vi "系统设置.vi"() -> ()   [LabVIEW 2016]
uses:
  <vilib>/Utility/miscctls.llb/LVPointTypeDef.ctl
  <vilib>/ptbypt/NI_PtbyPt.lvlib
  <vilib>/Utility/config.llb/NI_LVConfig.lvlib
  PLC/PLC.lvlib
panel:
  in  "更新":bool
  in  "updateconfiguration":T1={"主机"="27.154.58.30", "用户"="update", "密码"="std23506", "远程路径"="数据传输系统\\平台数据传输系统.exe", "下载文件名"="平台数据传输系统.exe", "软件版本"=""}
  in  "模块启用配置":bool
  in  "短信报警设置":bool
  in  "首页显示设置":bool
  in  "跨度核查":bool
  in  "空白核查":bool
  out "选项卡控件":enum32{"自由设定", "国标协议", "流量设定"}(tab)
  in  "24H周期设置":bool[](xcontrol)
  in  "运行间隔":i16=4 min=1 max=24
  in  "流量阈值":dbl=4.0 min=1.0 max=24.0
  in  "时间阈值":u16=4 min=1 max=24
  in  "周期设置":enum16{"自由设定", "国标协议", "流量设定"}(ring)
  out "x = y?":bool
  in  "质控启动日期":string(combo)="关闭"
  in  "跨度核查时间":u16(ring)=6 items=["00H", "01H", "02H", "03H", "04H", "05H", "06H", "07H", "08H", "09H", "10H", "11H", "12H", "13H", "14H", "15H", "16H", "17H", "18H", "19H", "20H", "21H", "22H", "23H", "关闭"]
  in  "空白核查时间":u16(ring)=2 items=["00H", "01H", "02H", "03H", "04H", "05H", "06H", "07H", "08H", "09H", "10H", "11H", "12H", "13H", "14H", "15H", "16H", "17H", "18H", "19H", "20H", "21H", "22H", "23H", "关闭"]
  in  "CODCr":bool
  in  "总磷总氮":bool
  in  "氨氮":bool
  in  "CODmn":bool
  in  "多参数":bool
  in  "输入密码":dbl
  in  "布尔":bool
  in  "副屏显示设置":bool
  in  "开机启动":bool caption="氨氮禁用"
  in  "运行模式":enum16{"维护模式", "常规模式", "应急模式", "质控模式"}(ring)
  # "注：周期设置分为自由设定和国标协议两种。\n1：选择自由设定情况下：运行间隔将不可选用并变灰色，周期设置可自由手动勾选\n2：选择国标协议情况下：周期时间将由运行间隔选择的时间决定，下方周期设置被禁用并无法手动勾选。\n3：选择流量设定情况下：瞬时流量连续超过流量阈值到达时间阈值设定值，仪器将自动开启测量。"
  # "自动运行启动参数"
  # "质控频次："
  # "空白核查时间："
  # "跨度核查时间："
  # "启动周期设置"
  # "m3/S"
  # "秒"
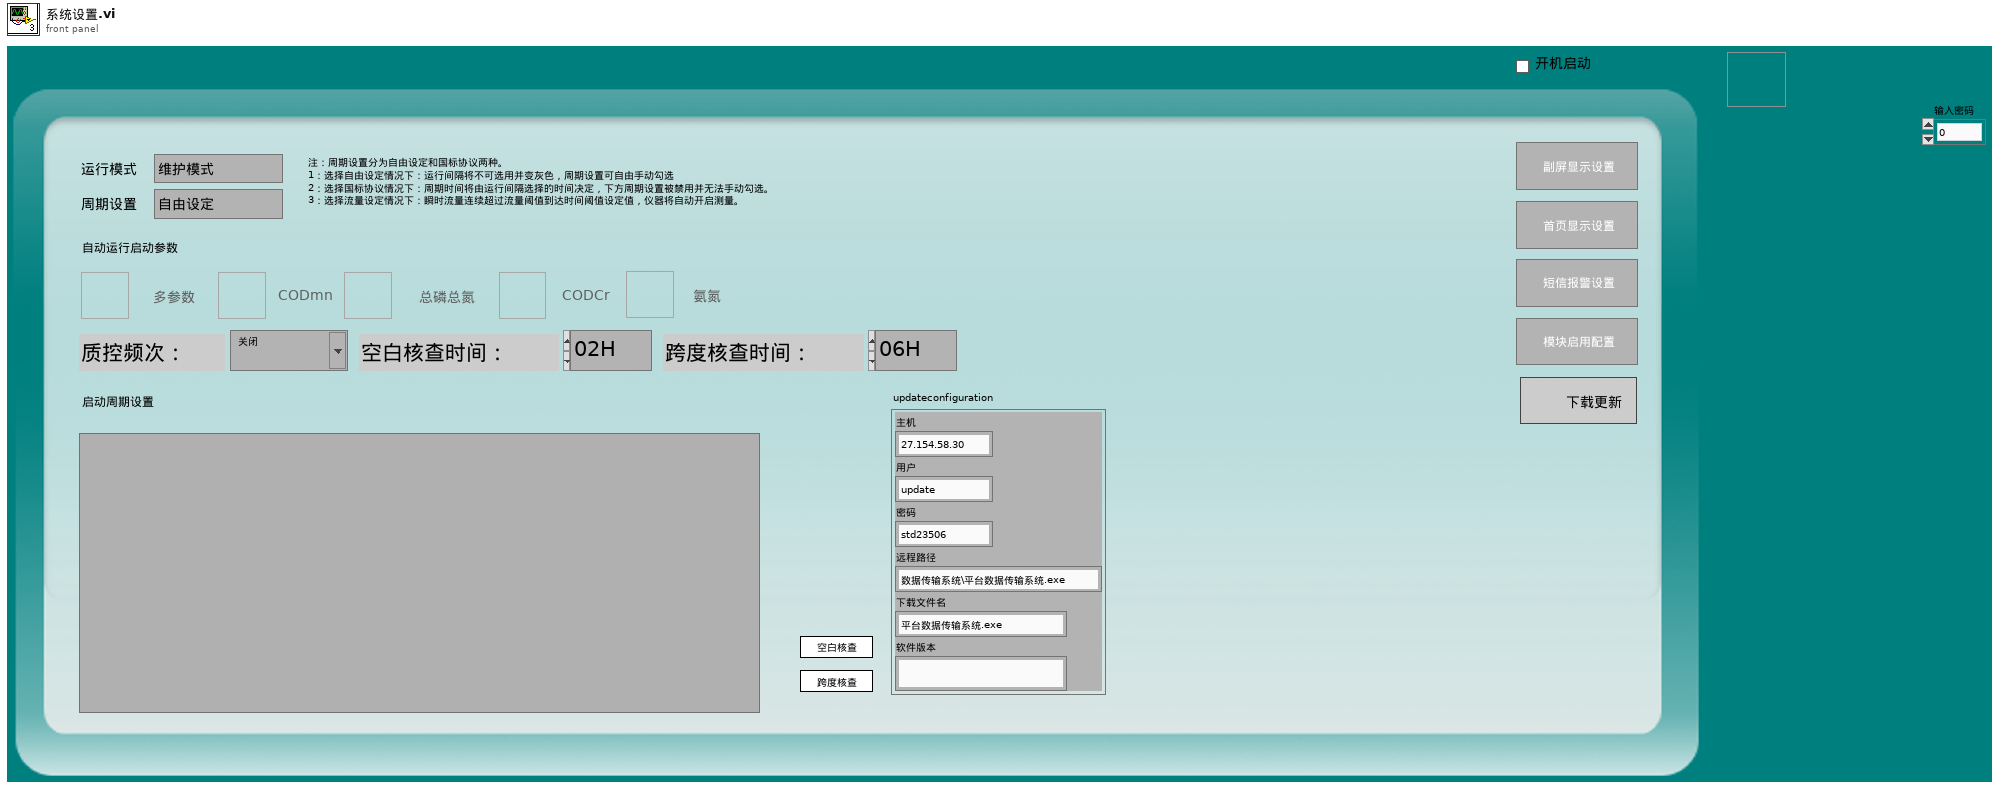
[diagram p1: front panel]
types:
  T1 = cluster{"主机":string, "用户":string, "密码":string, "远程路径":string, "下载文件名":string, "软件版本":string}
  T2 = typedef "NI_LVConfig.lvlib/Config Data RefNum.ctl" = refnum<k1>
  T3 = typedef "LVPointTypeDef.ctl" = cluster{"Horizontal":i16, "Vertical":i16}
  T4 = enum8{"Enabled", "Disabled", "Disabled and Grayed Out"}
  T5 = enum32{"Bad", "Idle", "Run top level", "Running"}
  T6 = enum32{"Invalid", "Standard", "Closed", "Hidden", "Minimized", "Maximized"}
  T7 = cluster{"运行模式":enum16{"维护模式", "常规模式", "应急模式", "质控模式"}}
  T8 = cluster{"测量模式":enum16{"水样测量", "标样核查", "零点核查", "跨度核查", "空白测试", "加标回收", "平行样", "校零", "校标"}}
  T9 = enum16{"启动测量", "标样核查", "零点核查", "跨度核查", "空白测试", "平行样测试", "加标回收", "空白校准", "标样校准", "初始化（清洗）", "停止测试", "仪器重启", "校时", "模式设置", "测量间隔设置"}
  T10 = cluster{"测试模式":enum16{"正常测试", "集成干预"}, "参数启用":cluster{"氨氮":bool, "总磷总氮":bool, "CODMn":bool, "CODcr":bool, "多参数":bool}}
  T11 = typedef "LVDateTimeRec.ctl" = cluster{"秒数的小数部分":dbl, "秒":i32, "分":i32, "时":i32, "日":i32, "月":i32, "年":i32, "天数（周）":i32, "天数（年）":i32, "DST":i32}
  T12 = cluster{"运行模式":enum16{"维护模式", "常规模式", "应急模式", "质控模式"}, "24H周期设置":bool[]}
  T13 = cluster{"运行模式":enum16{"维护模式", "常规模式", "应急模式", "质控模式"}, "质控频次":enum16{"关闭", "每天", "星期一", "星期二", "星期三", "星期四", "星期五", "星期六", "星期日"}, "空白核查时间":u16, "跨度核查时间":u16, "24H周期设置":bool[]}
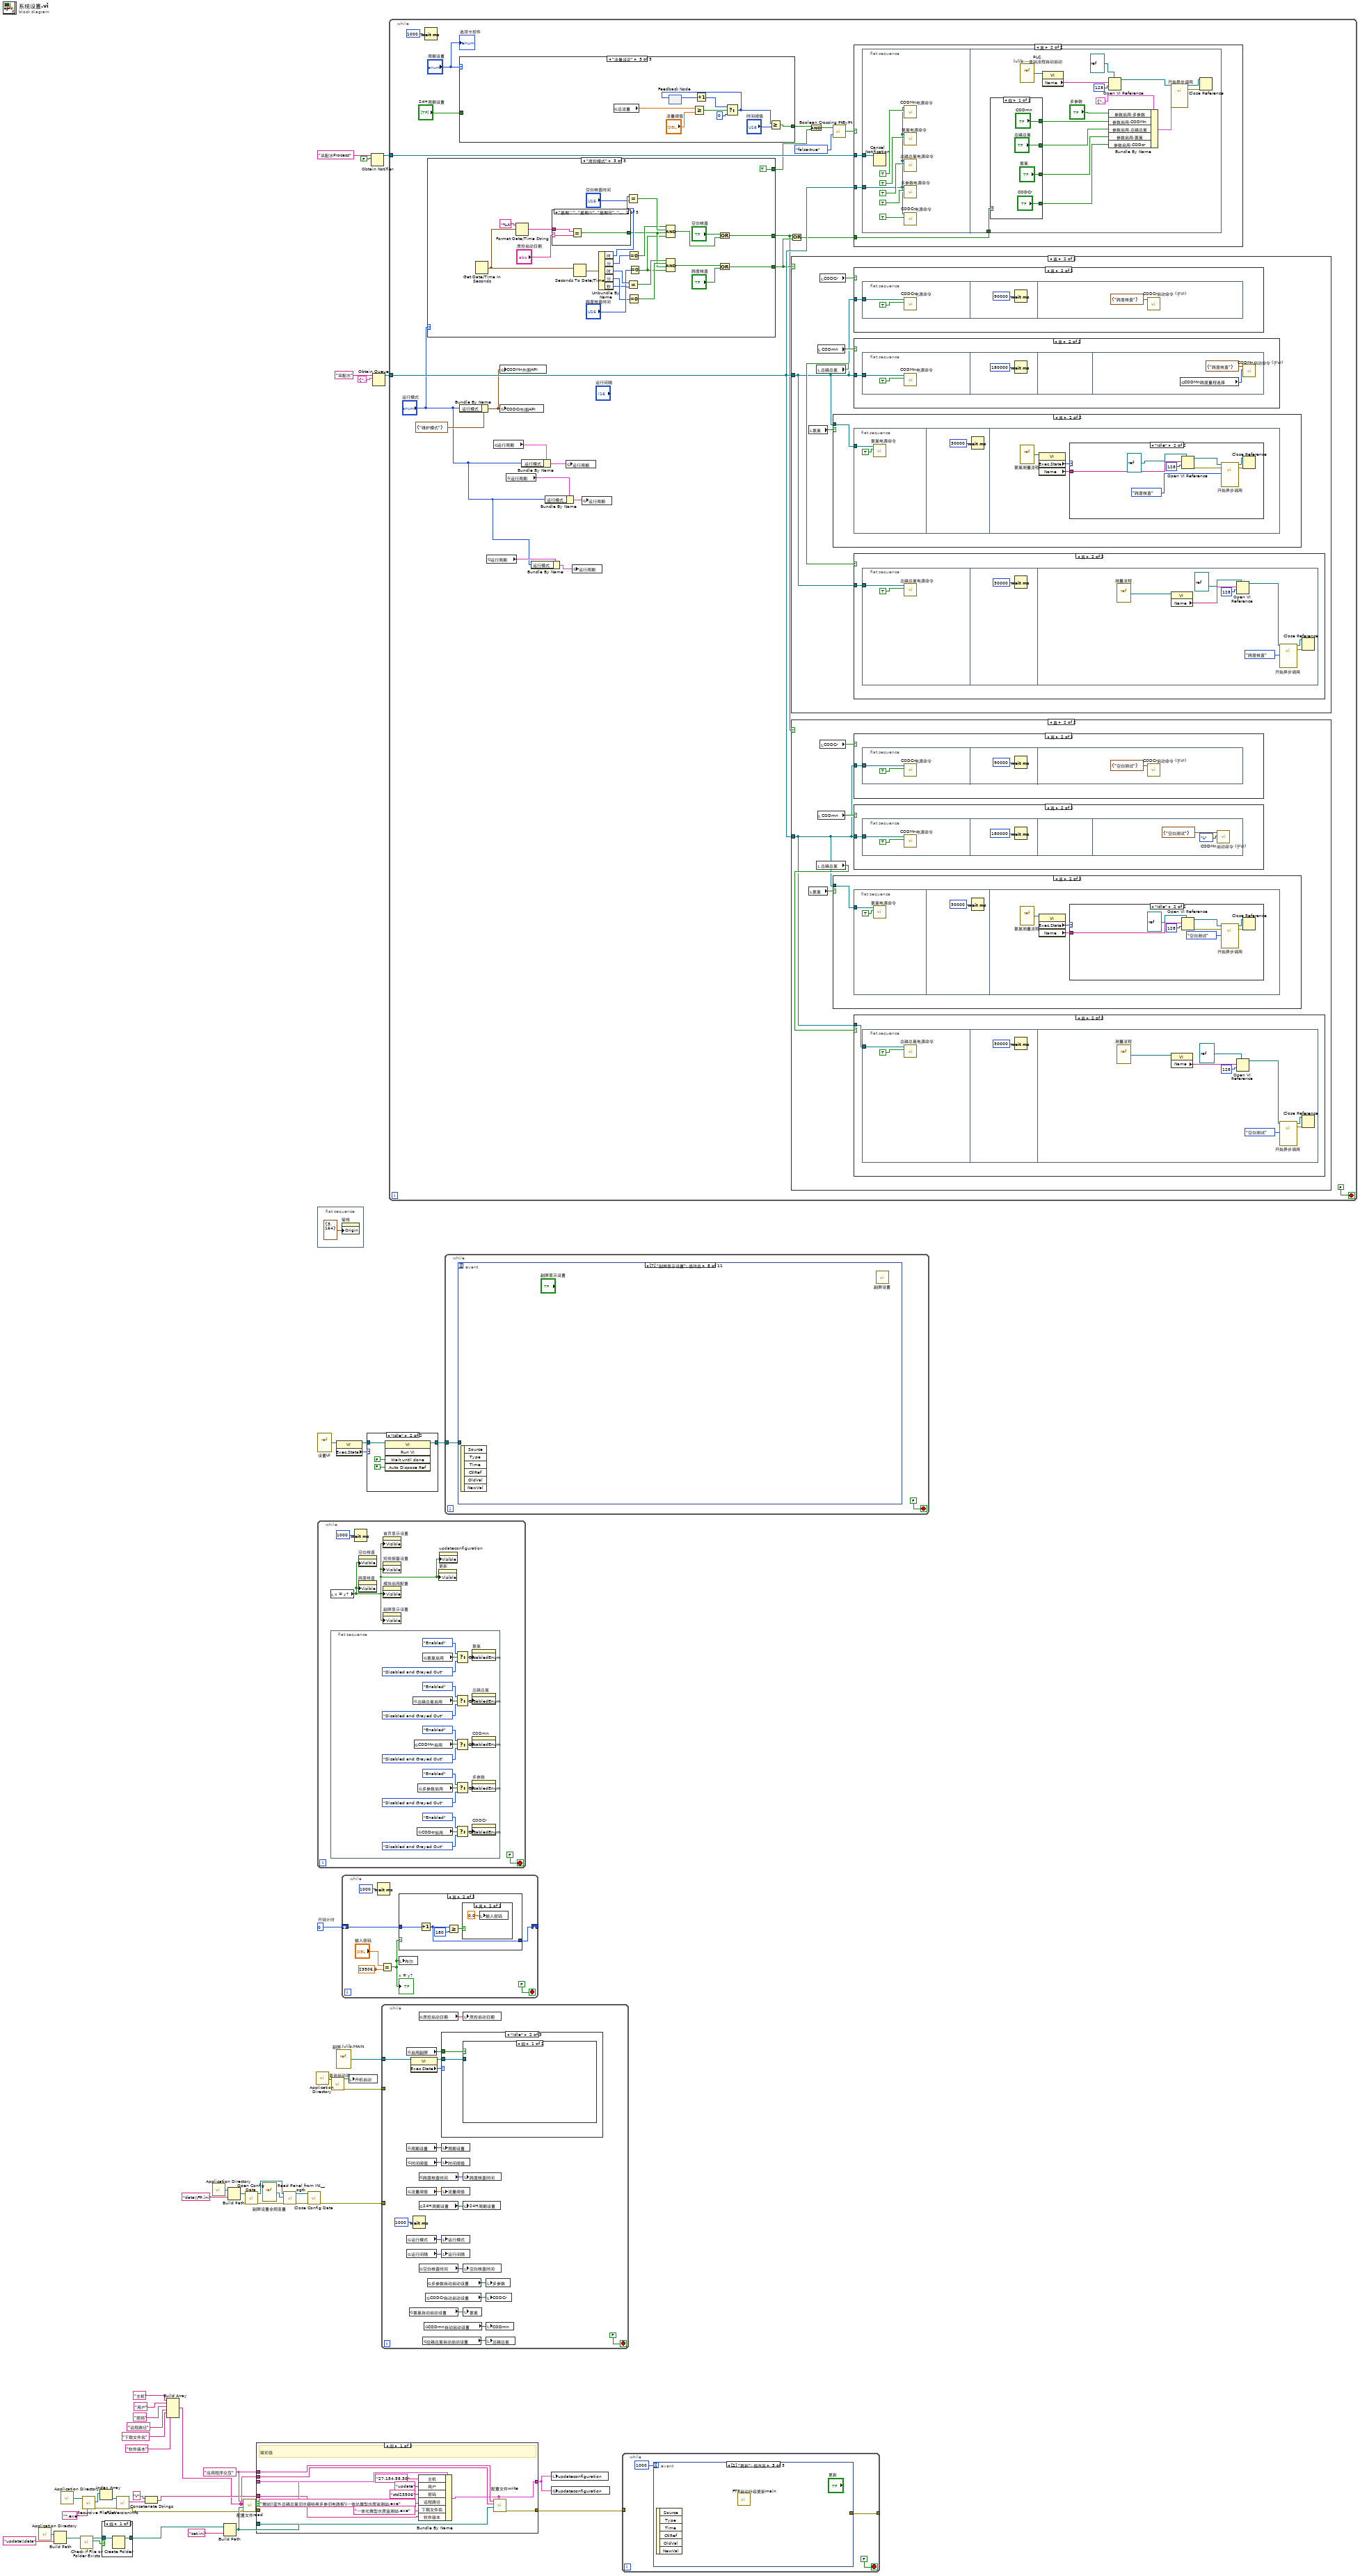
[diagram p0: block diagram]
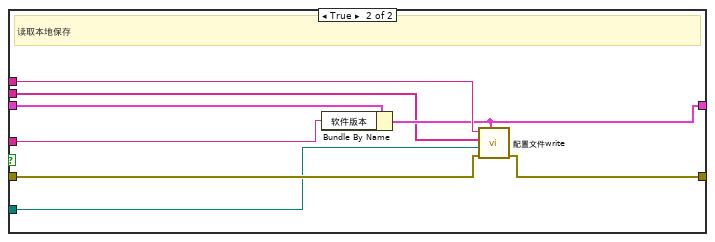
[diagram p3: hidden frame]
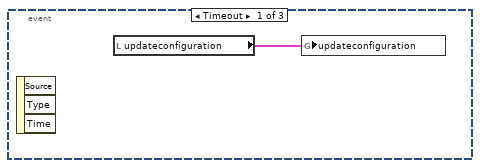
[diagram p4: hidden frame]
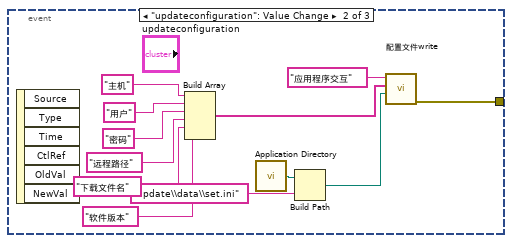
[diagram p5: hidden frame]
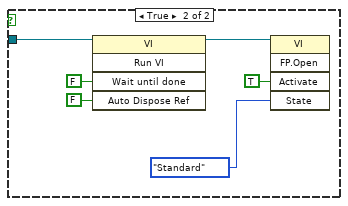
[diagram p10: hidden frame]
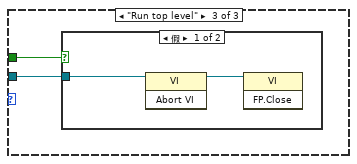
[diagram p11: hidden frame]
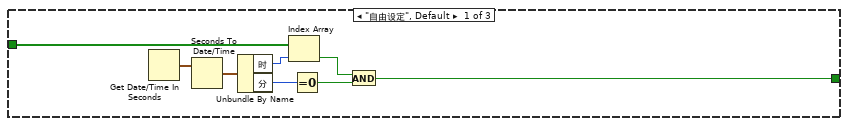
[diagram p13: hidden frame]
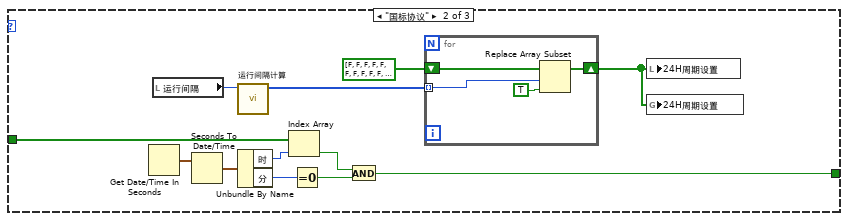
[diagram p14: hidden frame]
diagram:
  w28 = "应用程序交互" ("section")
  w49 = u32 0  # 开锁计时
  n1 = call <vilib>:"Application Directory.vi"() -> ("Application Directory"=w5:path)
  n2 = Build Path(base path=w5, name or relative path="update\\data" ("名称或相对路径")) -> (appended path=w6:path)
  n3 = call <vilib>:"Application Directory.vi"() -> ("Application Directory"=w23:path)
  n4 = call <vilib>:"Check if File or Folder Exists.vi"("path"=w6) -> ("file or folder exists?"=w7:bool, "dup path"=w8:path)  [unwired: 8 in, 1 out]
  n5 = call <vilib>:"Recursive File List.vi"("pattern"="*.exe", "Folder Path"=w23) -> ("error out"=w20:errorcluster, "All Files in Dir"=w22:path[])  [unwired: 5 in, 3 out]
  n6 = Index Array(array=w22) -> (element=w24:path)  [unwired: 1 in]
  n7 = case shown="假" w7 {
    tunnel: w8 -> [w56 w57]
    tunnel: [w55 w57] -> w3
    frame False {
      n8 = Create Folder(path (use dialog)=w56) -> (created path=w55:path)  [unwired: 2 in, 2 out]
    }
    frame True {
    }
  }
  n9 = call <vilib>:"FileVersionInfo.vi"("error in (no error)"=w20, "Application Path in"=w24) -> ("error out"=w17:errorcluster, "File Version Info"=w18:string)  [unwired: 6 in, 2 out]
  n10 = Concatenate Strings("V" ("字符串"), w18) -> (w16:string)
  n11 = Build Array("主机" ("section"), "用户" ("section"), "密码" ("key"), "远程路径" ("key"), "下载文件名" ("key"), "软件版本" ("key")) -> (w2:string[])
  n12 = call <vilib>:"Application Directory.vi"() -> ("Application Directory"=w31:path)
  n13 = Build Path(base path=w3, name or relative path="set.ini" ("名称或相对路径")) -> (appended path=w27:path)
  n14 = Build Path(base path=w31, name or relative path="data\\FP.ini" ("名称或相对路径")) -> (appended path=w38:path)
  n15 = call "配置文件read.vi"("error in (no error)"=w17, "configuration file path"=w27, "键数组"=w2, "段"=w28) -> ("error out"=w26:errorcluster, "section exists?"=w29:bool, "updateconfiguration"=w25:T1)  [unwired: 5 in]
  n16 = call <vilib>:"Open Config Data.vi"("configuration file path"=w38) -> ("error out"=w37:errorcluster, "refnum"=w34:T2)  [unwired: 8 in, 1 out]
  n17 = case shown="假" w29 {
    tunnel: w2 -> [w69 w73]
    tunnel: w28 -> [w68 w77]
    tunnel: w27 -> [w67 w71]
    tunnel: w26 -> [_ w72]
    tunnel: [w66 w70] -> w15
    tunnel: w25 -> [w60 w76]
    tunnel: [w58 w74] -> w1
    tunnel: w16 -> [w59 w75]
    frame False {
      # "赋初值"
      n18 = Bundle By Name(cluster=w60, "主机"="27.154.58.30" ("key"), "用户"="update", "密码"="std23506", "远程路径"="微站\\室外总磷总氮旧水箱哈希多参旧电路板\\一体化微型水质监测站.exe", "下载文件名"="一体化微型水质监测站.exe", "软件版本"=w59) -> (w58:T1)
      n19 = call "配置文件write.vi"("updateconfiguration"=w58, "configuration file path"=w67, "键数组"=w69, "段"=w68) -> ("error out"=w66:errorcluster)  [unwired: 7 in]
    }
    frame True {
      # "读取本地保存"
      n20 = Bundle By Name(cluster=w76, "软件版本"=w75) -> (w74:T1)
      n21 = call "配置文件write.vi"("updateconfiguration"=w74, "error in (no error)"=w72, "configuration file path"=w71, "键数组"=w73, "段"=w77) -> ("error out"=w70:errorcluster)  [unwired: 6 in]
    }
  }
  n22 = vi-ref "副屏设置全局变量.vi"() -> (w35:refnum<vi>)
  n23 = call <userlib>:"Read Panel from INI__ogtk.vi"("error in (no error)"=w37, "VI ref"=w35, "refnum"=w34) -> ("error out"=w36:errorcluster, "refnum out"=w33:T2)  [unwired: 7 in]
  n24 = call <vilib>:"Close Config Data.vi"("error in (no error)"=w36, "refnum"=w33) -> ("error out"=w32:errorcluster)  [unwired: 8 in, 1 out]
  n25 = call <vilib>:"Application Directory.vi"() -> ("Application Directory"=w51:path)
  n26 = flat-sequence {
    frame #0 {
      n27 = property on="窗格" class="Pane"("Origin"=T3 {"Horizontal"=3, "Vertical"=164} ("原点")) -> ()  [unwired: 2 in, 2 out]
    }
  }
  n28 = vi-ref "设置UI.vi"() -> (w44:refnum<vi>)
  n29 = while {
    stop <- FALSE stop-if-true
    n30 = local read "x = y?"() -> (w79:bool)
    n31 = flat-sequence {
      frame #0 {
        n32 = global read "系统设置全局变量.vi" "总磷总氮启用"() -> (w89:bool)
        n33 = global read "系统设置全局变量.vi" "CODMn启用"() -> (w87:bool)
        n34 = global read "系统设置全局变量.vi" "CODcr启用"() -> (w88:bool)
        n35 = global read "系统设置全局变量.vi" "多参数启用"() -> (w86:bool)
        n36 = global read "系统设置全局变量.vi" "氨氮启用"() -> (w82:bool)
        n37 = Select(t=T4."Enabled" ("禁用"), s=w82, f=T4."Disabled and Grayed Out" ("禁用")) -> (s? t:f=w90:T4)
        n38 = Select(t=T4."Enabled" ("禁用"), s=w89, f=T4."Disabled and Grayed Out" ("禁用")) -> (s? t:f=w84:T4)
        n39 = Select(t=T4."Enabled" ("禁用"), s=w87, f=T4."Disabled and Grayed Out" ("禁用")) -> (s? t:f=w91:T4)
        n40 = Select(t=T4."Enabled" ("禁用"), s=w86, f=T4."Disabled and Grayed Out" ("禁用")) -> (s? t:f=w85:T4)
        n41 = Select(t=T4."Enabled" ("禁用"), s=w88, f=T4."Disabled and Grayed Out" ("禁用")) -> (s? t:f=w101:T4)
        n42 = property on="氨氮" class="Bool (严格)"("DisabledEnum"=w90) -> ()  [unwired: 2 in, 2 out]
        n43 = property on="总磷总氮" class="Bool (严格)"("DisabledEnum"=w84) -> ()  [unwired: 2 in, 2 out]
        n44 = property on="CODmn" class="Bool (严格)"("DisabledEnum"=w91) -> ()  [unwired: 2 in, 2 out]
        n45 = property on="多参数" class="Bool (严格)"("DisabledEnum"=w85) -> ()  [unwired: 2 in, 2 out]
        n46 = property on="CODCr" class="Bool (严格)"("DisabledEnum"=w101) -> ()  [unwired: 2 in, 2 out]
      }
    }
    n47 = Wait (ms)(milliseconds to wait=u32 1000 ("等待时间（毫秒）")) -> ()  [unwired: 1 out]
    n48 = property on="空白核查" class="Bool"("Visible"=w79) -> ()  [unwired: 2 in, 2 out]
    n49 = property on="跨度核查" class="Bool"("Visible"=w79) -> ()  [unwired: 2 in, 2 out]
    n50 = property on="首页显示设置" class="Bool"("Visible"=w79) -> ()  [unwired: 2 in, 2 out]
    n51 = property on="短信报警设置" class="Bool"("Visible"=w79) -> ()  [unwired: 2 in, 2 out]
    n52 = property on="模块启用配置" class="Bool"("Visible"=w79) -> ()  [unwired: 2 in, 2 out]
    n53 = property on="副屏显示设置" class="Bool"("Visible"=w79) -> ()  [unwired: 2 in, 2 out]
    n54 = property on="更新" class="Bool"("Visible"=w79) -> ()  [unwired: 2 in, 2 out]
    n55 = property on="updateconfiguration" class="Clust (严格)"("Visible"=w79) -> ()  [unwired: 2 in, 2 out]
  }
  n56 = call "查询启动项.vi"("启动文件路径"=w51) -> ("error out"=w40:errorcluster, "包含启动项"=w50:bool)  [unwired: 9 in]
  n57 = property class="VI"(reference=w44) -> (reference out=w42:refnum<vi>, "Exec.State"=w43:T5)  [unwired: 1 in, 1 out]
  n58 = vi-ref "副屏.lvlib:MAIN.vi"() -> (w45:refnum<vi>)
  n59 = while {
    shift-right: [w103] -> _
    shift-left: w49 -> [w104]
    stop <- FALSE stop-if-true
    n60 = Wait (ms)(milliseconds to wait=u32 1000 ("等待时间（毫秒）")) -> ()  [unwired: 1 out]
    n61 = Equal?(x="输入密码", y=23506.0) -> (x = y?=w102:bool)
    "x = y?" <- w102
    n62 = case shown="真" w102 {
      tunnel: w104 -> [_ w112]
      tunnel: [_ w111] -> w103
      frame False {
      }
      frame True {
        n63 = Increment(x=w112) -> (x+1=w111:u32)
        n64 = Greater Or Equal?(x=w111, y=u32 180) -> (x >= y?=w109:bool)
        n65 = case shown="真" w109 {
          frame False {
          }
          frame True {
            n66 = local write "输入密码"(0.0 ("输入密码")) -> ()
          }
        }
      }
    }
    n67 = local write "布尔"(w102) -> ()
  }
  n68 = local write "开机启动"(w50) -> ()
  n69 = case shown="\"Idle\"" w43 {
    tunnel: w42 -> [w114 w118]
    tunnel: [w114 w117] -> w41
    frame "Bad", Default {
    }
    frame "Idle" {
      n70 = invoke class="VI" method="Run VI"(reference=w118, "Wait until done"=FALSE ("结束前等待"), "Auto Dispose Ref"=FALSE ("自动销毁引用")) -> (reference out=w117:refnum<vi>)  [unwired: 2 in, 4 out]
    }
  }
  n71 = Obtain Notifier(name (unnamed)="采配水Process" ("名称（未命名）"), notification data type=FALSE) -> (notifier out=w52:refnum<notifier>)  [unwired: 2 in, 2 out]
  n72 = Obtain Queue(name (unnamed)="采配水" ("名称（未命名）"), element data type=cluster{"命令":string, "数据":variant} {"命令"="", "数据"=variant}) -> (queue out=w46:refnum<queue>)  [unwired: 3 in, 2 out]
  n73 = while {
    tunnel: w45 -> [w130]
    tunnel: w40 -> [_]
    tunnel: w32 -> [_]
    stop <- FALSE stop-if-true
    n74 = global read "副屏设置全局变量.vi" "启用副屏"() -> (w128:bool)
    n75 = global read "系统设置全局变量.vi" "周期设置"() -> (w123:enum16{"自由设定", "国标协议", "流量设定"})
    n76 = global read "系统设置全局变量.vi" "时间阈值"() -> (w119:u16)
    n77 = global read "系统设置全局变量.vi" "流量阈值"() -> (w120:dbl)
    n78 = global read "系统设置全局变量.vi" "运行模式"() -> (w121:enum16{"维护模式", "常规模式", "应急模式", "质控模式"})
    n79 = global read "系统设置全局变量.vi" "运行间隔"() -> (w122:i16)
    n80 = global read "系统设置全局变量.vi" "氨氮自动启动设置"() -> (w135:bool)
    n81 = property class="VI"(reference=w130) -> (reference out=w127:refnum<vi>, "Exec.State"=w129:T5)  [unwired: 1 in, 1 out]
    n82 = Wait (ms)(milliseconds to wait=u32 1000 ("等待时间（毫秒）")) -> ()  [unwired: 1 out]
    n83 = global read "系统设置全局变量.vi" "质控启动日期"() -> (w126:string)
    n84 = global read "系统设置全局变量.vi" "跨度核查时间"() -> (w124:u16)
    n85 = global read "系统设置全局变量.vi" "24H周期设置"() -> (w136:bool[])
    n86 = global read "系统设置全局变量.vi" "空白核查时间"() -> (w125:u16)
    n87 = global read "系统设置全局变量.vi" "总磷总氮自动启动设置"() -> (w133:bool)
    n88 = global read "系统设置全局变量.vi" "CODmn自动启动设置"() -> (w132:bool)
    n89 = global read "系统设置全局变量.vi" "CODCr自动启动设置"() -> (w134:bool)
    n90 = global read "系统设置全局变量.vi" "多参数自动启动设置"() -> (w131:bool)
    n91 = case shown="\"Idle\"" w129 {
      tunnel: w128 -> [_ w139 w147]
      tunnel: w127 -> [_ w140 w148]
      frame "Bad", Default {
      }
      frame "Idle" {
        n92 = case shown="假" w139 {
          tunnel: w140 -> [_ w146]
          frame False {
          }
          frame True {
            n93 = invoke class="VI" method="Run VI"(reference=w146, "Wait until done"=FALSE ("结束前等待"), "Auto Dispose Ref"=FALSE ("自动销毁引用")) -> (reference out=w141:refnum<vi>)  [unwired: 2 in, 4 out]
            n94 = invoke class="VI" method="FP.Open"(reference=w141, "Activate"=TRUE ("激活？"), "State"=T6."Standard" ("状态")) -> ()  [unwired: 2 in, 5 out]
          }
        }
      }
      frame "Run top level" {
        n95 = case shown="假" w147 {
          tunnel: w148 -> [w149 _]
          frame False {
            n96 = invoke class="VI" method="Abort VI"(reference=w149) -> (reference out=w150:refnum<vi>)  [unwired: 2 in, 2 out]
            n97 = invoke class="VI" method="FP.Close"(reference=w150) -> ()  [unwired: 2 in, 3 out]
          }
          frame True {
          }
        }
      }
    }
    n98 = local write "周期设置"(w123) -> ()
    n99 = local write "时间阈值"(w119) -> ()
    n100 = local write "流量阈值"(w120) -> ()
    n101 = local write "运行模式"(w121) -> ()
    n102 = local write "运行间隔"(w122) -> ()
    n103 = local write "质控启动日期"(w126) -> ()
    n104 = local write "跨度核查时间"(w124) -> ()
    n105 = local write "24H周期设置"(w136) -> ()
    n106 = local write "空白核查时间"(w125) -> ()
    n107 = local write "氨氮"(w135) -> ()
    n108 = local write "多参数"(w131) -> ()
    n109 = local write "CODCr"(w134) -> ()
    n110 = local write "CODmn"(w132) -> ()
    n111 = local write "总磷总氮"(w133) -> ()
  }
  n112 = while {
    tunnel: w52 -> [w171]
    tunnel: w46 -> [w167]
    stop <- FALSE stop-if-true
    n113 = Wait (ms)(milliseconds to wait=u32 1000 ("等待时间（毫秒）")) -> ()  [unwired: 1 out]
    n114 = case shown="\"质控模式\"" "运行模式" {
      tunnel: [_ _ w323] -> w161
      tunnel: [_ _ w327] -> w160
      tunnel: [_ TRUE TRUE] -> w164
      frame "维护模式", Default {
      }
      frame "常规模式" {
      }
      frame "质控模式" {
        n115 = Get Date/Time In Seconds() -> (seconds since 1Jan1904=w334:timestamp)
        n116 = Format Date/Time String(time format string (%c)="%A" ("时间格式字符串(%c)"), seconds (now)=w334) -> (date/time string=w332:string)  [unwired: 1 in]
        n117 = case shown="\"星期二\", \"星期六\", \"星期日\", \"星期三\", \"星期四\", \"星期五\", \"星期一\"" "质控启动日期" {
          selector: "质控启动日期" -> [w350 _ _]
          tunnel: [w349 TRUE FALSE] -> w335
          tunnel: w332 -> [w348 _ _]
          frame "星期二", "星期六", "星期日", "星期三", "星期四", "星期五", "星期一" {
            n118 = Equal?(x=w348, y=w350) -> (x = y?=w349:bool)
          }
          frame "每天" {
          }
          frame "关闭", Default {
          }
        }
        n119 = Seconds To Date/Time(time stamp (now)=w334) -> (date time rec=w347:T11)  [unwired: 1 in]
        n120 = Unbundle By Name(w347) -> ("时"=w346:i32, "分"=w344:i32, "时"=w340:i32, "分"=w339:i32, "秒"=w331:i32)
        n121 = Equal?(x=w346, y="空白核查时间") -> (x = y?=w343:bool)
        n122 = Equal?(x=w340, y="跨度核查时间") -> (x = y?=w338:bool)
        n123 = Equal To 0?(x=w344) -> (x = 0?=w342:bool)
        n124 = Equal To 0?(x=w339) -> (x = 0?=w337:bool)
        n125 = Equal To 0?(x=w331) -> (x = 0?=w330:bool)
        n126 = Compound Arithmetic op=AND ("复合运算")(w342, w343, w335, w330) -> (w328:bool)
        n127 = Compound Arithmetic op=AND ("复合运算")(w338, w337, w335, w330) -> (w325:bool)
        n128 = Or(x="空白核查", y=w328) -> (x .or. y?=w327:bool)
        n129 = Or(x=w325, y="跨度核查") -> (x .or. y?=w323:bool)
      }
    }
    n130 = case shown="\"流量设定\"" "周期设置" {
      tunnel: [w175 w182 w198] -> w163
      tunnel: "24H周期设置" -> [w174 w183 _]
      frame "自由设定", Default {
        n131 = Get Date/Time In Seconds() -> (seconds since 1Jan1904=w176:timestamp)
        n132 = Seconds To Date/Time(time stamp (now)=w176) -> (date time rec=w177:T11)  [unwired: 1 in]
        n133 = Unbundle By Name(w177) -> ("时"=w180:i32, "分"=w178:i32)
        n134 = Index Array(array=w174, index=w180) -> (element=w181:bool)
        n135 = Equal To 0?(x=w178) -> (x = 0?=w179:bool)
        n136 = And(x=w181, y=w179) -> (x .and. y?=w175:bool)
      }
      frame "国标协议" {
        n137 = Get Date/Time In Seconds() -> (seconds since 1Jan1904=w184:timestamp)
        n138 = local read "运行间隔"() -> (w193:i16)
        n139 = Seconds To Date/Time(time stamp (now)=w184) -> (date time rec=w185:T11)  [unwired: 1 in]
        n140 = call "运行间隔计算.vi"("运行周期"=w193) -> ("数组"=w192:i32[])  [unwired: 10 in]
        n141 = Unbundle By Name(w185) -> ("时"=w188:i32, "分"=w186:i32)
        n142 = Index Array(array=w183, index=w188) -> (element=w189:bool)
        n143 = Equal To 0?(x=w186) -> (x = 0?=w187:bool)
        n144 = And(x=w189, y=w187) -> (x .and. y?=w182:bool)
        n145 = for {
          tunnel: w192 -> [w196] mode=indexing
          shift-right: [w194] -> w190
          shift-left: bool[] [FALSE, FALSE, FALSE, FALSE, FALSE, FALSE, FALSE, FALSE, FALSE, FALSE, FALSE, FALSE, FALSE, FALSE, FALSE, FALSE, FALSE, FALSE, FALSE, FALSE, FALSE, FALSE, FALSE, FALSE] ("24H周期设置") -> [w197]
          n146 = Replace Array Subset(array=w197, new element=TRUE ("新元素/子数组"), index=w196) -> (w194:bool[])
        }
        n147 = local write "24H周期设置"(w190) -> ()
        n148 = global write "系统设置全局变量.vi" "24H周期设置"(w190) -> ()
      }
      frame "流量设定" {
        n149 = global read "流量计全局变量.vi" "总流量"() -> (w206:dbl)
        n150 = feedback #1() -> (w203:i16)  [unwired: 1 in]
        n151 = Greater Or Equal?(x=w206, y="流量阈值") -> (x >= y?=w201:bool)
        n152 = Increment(x=w203) -> (x+1=w202:i16)
        n153 = Select(t=w202, s=w201, f=i16 0) -> (s? t:f=w200:i16)
        n154 = feedback-in #1(w200) -> ()
        n155 = Greater Or Equal?(x=w200, y="时间阈值") -> (x >= y?=w198:bool)
      }
    }
    n156 = Bundle By Name(cluster=T7 {"运行模式"=enum."维护模式"} ("外围API"), "运行模式"="运行模式") -> (w158:T7)
    n157 = global read "多参数断电保存全局变量.vi" "运行周期"() -> (w153:T12)
    n158 = global read "总磷总氮断电保存全局变量.vi" "运行周期"() -> (w157:T13)
    n159 = global write "CODMN外部API.vi" "CODMn外围API"(w158) -> ()
    n160 = global write "CODCr外部API.vi" "CODCr外围API"(w158) -> ()
    n161 = global read "氨氮断电保存全局变量.vi" "运行周期"() -> (w155:T13)
    n162 = Bundle By Name(cluster=w157, "运行模式"="运行模式") -> (w156:T13)
    n163 = Bundle By Name(cluster=w153, "运行模式"="运行模式") -> (w151:T12)
    n164 = Bundle By Name(cluster=w155, "运行模式"="运行模式") -> (w154:T13)
    n165 = global write "总磷总氮断电保存全局变量.vi" "运行周期"(w156) -> ()
    n166 = global write "多参数断电保存全局变量.vi" "运行周期"(w151) -> ()
    n167 = global write "氨氮断电保存全局变量.vi" "运行周期"(w154) -> ()
    n168 = Or(x=w160, y=w161) -> (x .or. y?=w159:bool)
    n169 = case shown="真" w161 {
      tunnel: w167 -> [_ w207]
      frame False {
      }
      frame True {
        n170 = local read "氨氮"() -> (w211:bool)
        n171 = local read "总磷总氮"() -> (w210:bool)
        n172 = local read "CODmn"() -> (w209:bool)
        n173 = local read "CODCr"() -> (w208:bool)
        n174 = case shown="真" w211 {
          tunnel: w207 -> [_ w235]
          frame False {
          }
          frame True {
            n175 = flat-sequence {
              tunnel: w235 -> [w236]
              frame #0 {
                n176 = call "氨氮电源命令.vi"("通电/断电"=TRUE, "队列"=w236) -> ()  [unwired: 9 in, 1 out]
              }
              frame #1 {
                n177 = Wait (ms)(milliseconds to wait=u32 30000 ("等待时间（毫秒）")) -> ()  [unwired: 1 out]
              }
              frame #2 {
                n178 = vi-ref "氨氮测量流程.vi"() -> (w241:refnum<vi>)
                n179 = property class="VI"(reference=w241) -> ("Exec.State"=w239:T5, "Name"=w240:string)  [unwired: 1 in, 2 out]
                n180 = case shown="\"Idle\"" w239 {
                  tunnel: w240 -> [_ w246]
                  frame "Bad", Default {
                  }
                  frame "Idle" {
                    n181 = Open VI Reference(type specifier VI Refnum (for type only)=refnum<vi> refnum, vi path=w246, options=128 ("选项")) -> (vi reference=w244:refnum<vi>, error out=w247:errorcluster)  [unwired: 3 in]
                    n182 = call-by-ref "开始异步调用"(reference=w244, error in=w247, "控制命令"=T9."跨度核查") -> (reference out=w248:refnum<vi>, error out=w249:errorcluster)  [unwired: 11 in]
                    n183 = Close Reference(reference=w248, error in (no error)=w249) -> ()  [unwired: 1 out]
                  }
                }
              }
            }
          }
        }
        n184 = case shown="真" w208 {
          tunnel: w207 -> [_ w212]
          frame False {
          }
          frame True {
            n185 = flat-sequence {
              tunnel: w212 -> [w213]
              frame #0 {
                n186 = call "CODCr电源命令.vi"("通电/断电"=TRUE, "队列"=w213) -> ()  [unwired: 9 in, 1 out]
              }
              frame #1 {
                n187 = Wait (ms)(milliseconds to wait=u32 90000 ("等待时间（毫秒）")) -> ()  [unwired: 1 out]
              }
              frame #2 {
                n188 = call "CODCr启动命令 (子VI).vi"("启动测量模式"=T8 {"测量模式"=enum."跨度核查"}) -> ()  [unwired: 11 in]
              }
            }
          }
        }
        n189 = case shown="真" w209 {
          tunnel: w207 -> [_ w217]
          frame False {
          }
          frame True {
            n190 = flat-sequence {
              tunnel: w217 -> [w218]
              frame #0 {
                n191 = call "CODMn电源命令.vi"("通电/断电"=TRUE, "队列"=w218) -> ()  [unwired: 9 in, 1 out]
              }
              frame #1 {
                n192 = Wait (ms)(milliseconds to wait=u32 180000 ("等待时间（毫秒）")) -> ()  [unwired: 1 out]
              }
              frame #2 {
              }
              frame #3 {
                n193 = global read "CODMn断电保存全局变量.vi" "CODMn跨度量程选择"() -> (w221:enum32{"H", "L", "AUTO"})
                n194 = call "CODMn启动命令 (子VI).vi"("CODMn量程切换"=w221, "启动测量模式"=T8 {"测量模式"=enum."跨度核查"}) -> ()  [unwired: 10 in]
              }
            }
          }
        }
        n195 = case shown="真" w210 {
          tunnel: w207 -> [_ w223]
          frame False {
          }
          frame True {
            n196 = flat-sequence {
              tunnel: w223 -> [w225]
              frame #0 {
                n197 = call "总磷总氮电源命令.vi"("通电/断电"=TRUE, "队列"=w225) -> ()  [unwired: 9 in, 1 out]
              }
              frame #1 {
                n198 = Wait (ms)(milliseconds to wait=u32 30000 ("等待时间（毫秒）")) -> ()  [unwired: 1 out]
              }
              frame #2 {
                n199 = vi-ref "测量流程.vi"() -> (w232:refnum<vi>)
                n200 = property class="VI"(reference=w232) -> ("Name"=w233:string)  [unwired: 1 in, 2 out]
                n201 = Open VI Reference(type specifier VI Refnum (for type only)=refnum<vi> refnum, vi path=w233, options=128 ("选项")) -> (vi reference=w231:refnum<vi>)  [unwired: 3 in, 1 out]
                n202 = call-by-ref "开始异步调用"(reference=w231, "控制命令"=T9."跨度核查") -> (reference out=w230:refnum<vi>, error out=w229:errorcluster)  [unwired: 12 in]
                n203 = Close Reference(reference=w230, error in (no error)=w229) -> ()  [unwired: 1 out]
              }
            }
          }
        }
      }
    }
    n204 = case shown="真" w160 {
      tunnel: w167 -> [_ w250]
      frame False {
      }
      frame True {
        n205 = local read "氨氮"() -> (w254:bool)
        n206 = local read "总磷总氮"() -> (w253:bool)
        n207 = local read "CODmn"() -> (w252:bool)
        n208 = local read "CODCr"() -> (w251:bool)
        n209 = case shown="真" w254 {
          tunnel: w250 -> [_ w278]
          frame False {
          }
          frame True {
            n210 = flat-sequence {
              tunnel: w278 -> [w279]
              frame #0 {
                n211 = call "氨氮电源命令.vi"("通电/断电"=TRUE, "队列"=w279) -> ()  [unwired: 9 in, 1 out]
              }
              frame #1 {
                n212 = Wait (ms)(milliseconds to wait=u32 30000 ("等待时间（毫秒）")) -> ()  [unwired: 1 out]
              }
              frame #2 {
                n213 = vi-ref "氨氮测量流程.vi"() -> (w284:refnum<vi>)
                n214 = property class="VI"(reference=w284) -> ("Exec.State"=w282:T5, "Name"=w283:string)  [unwired: 1 in, 2 out]
                n215 = case shown="\"Idle\"" w282 {
                  tunnel: w283 -> [_ w289]
                  frame "Bad", Default {
                  }
                  frame "Idle" {
                    n216 = Open VI Reference(type specifier VI Refnum (for type only)=refnum<vi> refnum, vi path=w289, options=128 ("选项")) -> (vi reference=w287:refnum<vi>, error out=w290:errorcluster)  [unwired: 3 in]
                    n217 = call-by-ref "开始异步调用"(reference=w287, error in=w290, "控制命令"=T9."空白测试") -> (reference out=w291:refnum<vi>, error out=w292:errorcluster)  [unwired: 11 in]
                    n218 = Close Reference(reference=w291, error in (no error)=w292) -> ()  [unwired: 1 out]
                  }
                }
              }
            }
          }
        }
        n219 = case shown="真" w251 {
          tunnel: w250 -> [_ w255]
          frame False {
          }
          frame True {
            n220 = flat-sequence {
              tunnel: w255 -> [w256]
              frame #0 {
                n221 = call "CODCr电源命令.vi"("通电/断电"=TRUE, "队列"=w256) -> ()  [unwired: 9 in, 1 out]
              }
              frame #1 {
                n222 = Wait (ms)(milliseconds to wait=u32 90000 ("等待时间（毫秒）")) -> ()  [unwired: 1 out]
              }
              frame #2 {
                n223 = call "CODCr启动命令 (子VI).vi"("启动测量模式"=T8 {"测量模式"=enum."空白测试"}) -> ()  [unwired: 11 in]
              }
            }
          }
        }
        n224 = case shown="真" w252 {
          tunnel: w250 -> [_ w260]
          frame False {
          }
          frame True {
            n225 = flat-sequence {
              tunnel: w260 -> [w261]
              frame #0 {
                n226 = call "CODMn电源命令.vi"("通电/断电"=TRUE, "队列"=w261) -> ()  [unwired: 9 in, 1 out]
              }
              frame #1 {
                n227 = Wait (ms)(milliseconds to wait=u32 180000 ("等待时间（毫秒）")) -> ()  [unwired: 1 out]
              }
              frame #2 {
              }
              frame #3 {
                n228 = call "CODMn启动命令 (子VI).vi"("CODMn量程切换"=enum32{"H", "L", "AUTO"}."L", "启动测量模式"=T8 {"测量模式"=enum."空白测试"}) -> ()  [unwired: 10 in]
              }
            }
          }
        }
        n229 = case shown="真" w253 {
          tunnel: w250 -> [_ w266]
          frame False {
          }
          frame True {
            n230 = flat-sequence {
              tunnel: w266 -> [w268]
              frame #0 {
                n231 = call "总磷总氮电源命令.vi"("通电/断电"=TRUE, "队列"=w268) -> ()  [unwired: 9 in, 1 out]
              }
              frame #1 {
                n232 = Wait (ms)(milliseconds to wait=u32 30000 ("等待时间（毫秒）")) -> ()  [unwired: 1 out]
              }
              frame #2 {
                n233 = vi-ref "测量流程.vi"() -> (w275:refnum<vi>)
                n234 = property class="VI"(reference=w275) -> ("Name"=w276:string)  [unwired: 1 in, 2 out]
                n235 = Open VI Reference(type specifier VI Refnum (for type only)=refnum<vi> refnum, vi path=w276, options=128 ("选项")) -> (vi reference=w274:refnum<vi>)  [unwired: 3 in, 1 out]
                n236 = call-by-ref "开始异步调用"(reference=w274, "控制命令"=T9."空白测试") -> (reference out=w273:refnum<vi>, error out=w272:errorcluster)  [unwired: 12 in]
                n237 = Close Reference(reference=w273, error in (no error)=w272) -> ()  [unwired: 1 out]
              }
            }
          }
        }
      }
    }
    n238 = And(x=w163, y=w164) -> (x .and. y?=w162:bool)
    n239 = call <vilib>:"Boolean Crossing PtByPt.vi"("direction"=enum16{"either", "false-true", "true-false"}."false-true", "input"=w162) -> ("crossing"=w169:bool)  [unwired: 1 in]
    n240 = case shown="真" w169 {
      tunnel: w171 -> [_ w295]
      tunnel: w167 -> [_ w294]
      tunnel: w159 -> [_ w293]
      frame False {
      }
      frame True {
        n241 = flat-sequence {
          tunnel: w295 -> [w302]
          tunnel: w294 -> [w296]
          tunnel: w293 -> [w306]
          frame #0 {
            n242 = Cancel Notification(0:w302) -> ()  [unwired: 1 in, 3 out]
            n243 = call "CODMn电源命令.vi"("通电/断电"=TRUE, "队列"=w296) -> ()  [unwired: 9 in, 1 out]
            n244 = call "氨氮电源命令.vi"("通电/断电"=TRUE, "队列"=w296) -> ()  [unwired: 9 in, 1 out]
            n245 = call "总磷总氮电源命令.vi"("通电/断电"=TRUE, "队列"=w296) -> ()  [unwired: 9 in, 1 out]
            n246 = call "多参数电源命令.vi"("通电/断电"=TRUE, "队列"=w296) -> ()  [unwired: 9 in, 1 out]
            n247 = call "CODCr电源命令.vi"("通电/断电"=TRUE, "队列"=w296) -> ()  [unwired: 9 in, 1 out]
          }
          frame #1 {
            n248 = case shown="假" w306 {
              tunnel: ["CODmn" _] -> w316
              tunnel: ["总磷总氮" _] -> w315
              tunnel: ["CODCr" _] -> w314
              tunnel: ["氨氮" _] -> w313
              frame False {
              }
              frame True {
              }
            }
            n249 = vi-ref "PLC.lvlib:一体站流程自动启动.vi"() -> (w310:refnum<vi>)
            n250 = property class="VI"(reference=w310) -> ("Name"=w311:string)  [unwired: 1 in, 2 out]
            n251 = Bundle By Name(cluster=T10 {"测试模式"=enum."正常测试", "参数启用"={"氨氮"=FALSE, "总磷总氮"=FALSE, "CODMn"=FALSE, "CODcr"=FALSE, "多参数"=FALSE}} ("参数"), "参数启用.多参数"="多参数", "参数启用.CODMn"=w316, "参数启用.总磷总氮"=w315, "参数启用.氨氮"=w313, "参数启用.CODcr"=w314) -> (w303:T10)
            n252 = Open VI Reference(type specifier VI Refnum (for type only)=refnum<vi> refnum, vi path=w311, options=128 ("选项")) -> (vi reference=w309:refnum<vi>)  [unwired: 3 in, 1 out]
            n253 = call-by-ref "开始异步调用"(reference=w309, "参数"=w303) -> (reference out=w308:refnum<vi>, error out=w307:errorcluster)  [unwired: 12 in]
            n254 = Close Reference(reference=w308, error in (no error)=w307) -> ()  [unwired: 1 out]
          }
        }
      }
    }
    "选项卡控件" <- "周期设置"
  }
  n255 = while {
    tunnel: w41 -> [w353]
    stop <- FALSE stop-if-true
    n256 = event shown="[7] \"副屏显示设置\": 值改变" {
      selector: _ -> [_ _ _ _ _ _ _ _ _ _ _]
      dyn-events: _ -> [_ _ _ _ _ _ _ _ _ _ _]
      timeout: _ -> [_ _ _ _ _ _ _ _ _ _ _]
      tunnel: w353 -> [_ _ _ _ _ _ _ _ _ w407 _]
      event Timeout {
        n257 = event-data() -> ()  [unwired: 1 in, 3 out]
      }
      event "模块启用配置": Value Change {
        n258 = event-data() -> ()  [unwired: 1 in, 6 out]
        n259 = call "模块启用配置框.vi"() -> ()  [unwired: 12 in]
      }
      event "24H周期设置", "运行模式", "多参数", "CODmn", "氨氮", "总磷总氮", "CODCr", "质控启动日期", "空白核查时间", "跨度核查时间", "运行间隔", "周期设置", "流量阈值", "时间阈值": Value Change {
        n260 = event-data() -> ()  [unwired: 1 in, 6 out]
        n261 = flat-sequence {
          frame #0 {
            n262 = local read "氨氮"() -> (w367:bool)
            n263 = local read "运行间隔"() -> (w358:i16)
            n264 = local read "流量阈值"() -> (w355:dbl)
            n265 = local read "总磷总氮"() -> (w365:bool)
            n266 = local read "周期设置"() -> (w357:enum16{"自由设定", "国标协议", "流量设定"})
            n267 = local read "时间阈值"() -> (w356:u16)
            n268 = local read "运行模式"() -> (w368:enum16{"维护模式", "常规模式", "应急模式", "质控模式"})
            n269 = local read "CODmn"() -> (w364:bool)
            n270 = local read "CODCr"() -> (w366:bool)
            n271 = local read "多参数"() -> (w363:bool)
            n272 = local read "空白核查时间"() -> (w360:u16)
            n273 = local read "质控启动日期"() -> (w361:string)
            n274 = local read "24H周期设置"() -> (w362:bool[])
            n275 = local read "跨度核查时间"() -> (w359:u16)
            n276 = global write "系统设置全局变量.vi" "氨氮自动启动设置"(w367) -> ()
            n277 = global write "系统设置全局变量.vi" "运行间隔"(w358) -> ()
            n278 = global write "系统设置全局变量.vi" "流量阈值"(w355) -> ()
            n279 = global write "系统设置全局变量.vi" "CODCr自动启动设置"(w366) -> ()
            n280 = global write "系统设置全局变量.vi" "总磷总氮自动启动设置"(w365) -> ()
            n281 = global write "系统设置全局变量.vi" "周期设置"(w357) -> ()
            n282 = global write "系统设置全局变量.vi" "CODmn自动启动设置"(w364) -> ()
            n283 = global write "系统设置全局变量.vi" "时间阈值"(w356) -> ()
            n284 = global write "系统设置全局变量.vi" "多参数自动启动设置"(w363) -> ()
            n285 = global write "系统设置全局变量.vi" "运行模式"(w368) -> ()
            n286 = global write "系统设置全局变量.vi" "空白核查时间"(w360) -> ()
            n287 = global write "系统设置全局变量.vi" "质控启动日期"(w361) -> ()
            n288 = global write "系统设置全局变量.vi" "24H周期设置"(w362) -> ()
            n289 = global write "系统设置全局变量.vi" "跨度核查时间"(w359) -> ()
          }
          frame #1 {
            n290 = call <vilib>:"Application Directory.vi"() -> ("Application Directory"=w382:path)
            n291 = Build Path(base path=w382, name or relative path="data\\sys.ini" ("名称或相对路径")) -> (appended path=w380:path)
            n292 = call <vilib>:"Open Config Data.vi"("configuration file path"=w380) -> ("error out"=w376:errorcluster, "refnum"=w379:T2)  [unwired: 8 in, 1 out]
            n293 = vi-ref "系统设置全局变量.vi"() -> (w378:refnum<vi>)
            n294 = call <userlib>:"Write Panel to INI__ogtk.vi"("error in (no error)"=w376, "VI ref"=w378, "refnum"=w379) -> ("error out"=w375:errorcluster, "refnum out"=w377:T2)  [unwired: 7 in]
            n295 = call <vilib>:"Close Config Data.vi"("error in (no error)"=w375, "refnum"=w377) -> ("error out"=w370:errorcluster, "file path"=w369:path)  [unwired: 8 in]
            n296 = Open/Create/Replace File(file path (use dialog)=w369, error in=w370) -> (refnum out=w373:refnum<file>, error out=w374:errorcluster)  [unwired: 4 in, 1 out]
            n297 = Flush File(refnum=w373, error in=w374) -> (refnum out=w372:refnum<file>, error out=w371:errorcluster)
            n298 = Close File(refnum=w372, error in=w371) -> ()  [unwired: 2 out]
          }
        }
      }
      event "运行间隔": Mouse Down {
        n299 = event-data() -> ("CtlRef"=w386:refnum<vi>)  [unwired: 1 in, 7 out]
        n300 = property class="DigNum (严格)"(reference=w386) -> (reference out=w385:refnum<vi>, "Value"=w384:i16)  [unwired: 1 in, 1 out]
        n301 = call "数字键盘.vi"("OldNumber"=w384) -> ("NewNumber"=w383:sgl)
        n302 = property class="DigNum (严格)"(reference=w385, "Val(Sgnl)"=w383) -> ()  [unwired: 1 in, 2 out]
      }
      event "流量阈值": Mouse Down {
        n303 = event-data() -> ("CtlRef"=w390:refnum<vi>)  [unwired: 1 in, 7 out]
        n304 = property class="DigNum (严格)"(reference=w390) -> (reference out=w389:refnum<vi>, "Value"=w388:dbl)  [unwired: 1 in, 1 out]
        n305 = call "数字键盘.vi"("OldNumber"=w388) -> ("NewNumber"=w387:sgl)
        n306 = property class="DigNum (严格)"(reference=w389, "Val(Sgnl)"=w387) -> ()  [unwired: 1 in, 2 out]
      }
      event "时间阈值": Mouse Down {
        n307 = event-data() -> ("CtlRef"=w394:refnum<vi>)  [unwired: 1 in, 7 out]
        n308 = property class="DigNum (严格)"(reference=w394) -> (reference out=w393:refnum<vi>, "Value"=w392:u16)  [unwired: 1 in, 1 out]
        n309 = call "数字键盘.vi"("OldNumber"=w392) -> ("NewNumber"=w391:sgl)
        n310 = property class="DigNum (严格)"(reference=w393, "Val(Sgnl)"=w391) -> ()  [unwired: 1 in, 2 out]
      }
      event "开机启动": Value Change {
        n311 = event-data() -> ("NewVal"=w396:bool)  [unwired: 1 in, 5 out]
        n312 = call <vilib>:"Application Directory.vi"() -> ("Application Directory"=w395:path)
        n313 = case shown="真" w396 {
          tunnel: w395 -> [w398 w402]
          frame False {
            n314 = call "删除启动项.vi"("启动文件路径"=w398) -> ("删除标记"=w397:bool)  [unwired: 9 in, 1 out]
            n315 = case shown="真" w397 {
              frame False {
                n316 = local write "开机启动"(TRUE ("开机启动")) -> ()
                n317 = One Button Dialog(message="启动项删除失败" ("消息")) -> ()  [unwired: 1 in, 1 out]
              }
              frame True {
              }
            }
          }
          frame True {
            n318 = call "添加启动项.vi"("启动文件路径"=w402) -> ("添加成功标记"=w401:bool)  [unwired: 9 in, 1 out]
            n319 = case shown="真" w401 {
              frame False {
                n320 = local write "开机启动"(FALSE ("开机启动")) -> ()
                n321 = One Button Dialog(message="启动项添加失败" ("消息")) -> ()  [unwired: 1 in, 1 out]
              }
              frame True {
              }
            }
          }
        }
      }
      event "副屏显示设置": Value Change {
        n322 = event-data() -> ()  [unwired: 1 in, 6 out]
        n323 = call "副屏设置.vi"() -> ()  [unwired: 12 in]
      }
      event "首页显示设置": Value Change {
        n324 = event-data() -> ()  [unwired: 1 in, 6 out]
        n325 = call "首页显示设置.vi"() -> ()  [unwired: 12 in]
      }
      event "短信报警设置": Value Change {
        n326 = event-data() -> ()  [unwired: 1 in, 6 out]
        n327 = invoke class="VI" method="FP.Open"(reference=w407, "Activate"=TRUE ("激活？"), "State"=T6."Standard" ("状态")) -> ()  [unwired: 2 in, 5 out]
      }
      event "布尔": Value Change {
        n328 = event-data() -> ("OldVal"=w409:bool)  [unwired: 1 in, 5 out]
        n329 = case shown="假" w409 {
          tunnel: [w410 _] -> w408
          frame False {
            n330 = call "数字密码键盘.vi"() -> ("NewNumber"=w410:sgl)  [unwired: 1 in]
          }
          frame True {
          }
        }
        n331 = local write "输入密码"(w408) -> ()
      }
    }
  }
  n332 = local write "updateconfiguration"(w1) -> ()
  n333 = global write "update全局.vi" "updateconfiguration"(w1) -> ()
  n334 = while {
    tunnel: [w411] -> _
    tunnel: w15 -> [_]
    stop <- FALSE stop-if-true
    n335 = event shown="[2] \"更新\": 值改变" {
      selector: _ -> [_ _ _]
      dyn-events: _ -> [_ _ _]
      timeout: 1000 -> [_ _ _]
      tunnel: [_ w422 _] -> w411
      event Timeout {
        n336 = event-data() -> ()  [unwired: 1 in, 3 out]
        n337 = local read "updateconfiguration"() -> (w414:T1)
        n338 = global write "update全局.vi" "updateconfiguration"(w414) -> ()
      }
      event "updateconfiguration": Value Change {
        n339 = event-data() -> ()  [unwired: 1 in, 6 out]
        n340 = Build Array("主机" ("section"), "用户" ("section"), "密码" ("key"), "远程路径" ("key"), "下载文件名" ("key"), "软件版本" ("key")) -> (w415:string[])
        n341 = call <vilib>:"Application Directory.vi"() -> ("Application Directory"=w425:path)
        n342 = Build Path(base path=w425, name or relative path="update\\data\\set.ini" ("名称或相对路径")) -> (appended path=w423:path)
        n343 = call "配置文件write.vi"("configuration file path"=w423, "键数组"=w415, "段"="应用程序交互" ("section")) -> ("error out"=w422:errorcluster)  [unwired: 8 in]
      }
      event "更新": Value Change {
        n344 = event-data() -> ()  [unwired: 1 in, 6 out]
        n345 = call "FTP自动升级更新main.vi"() -> ()  [unwired: 12 in]
      }
    }
  }
